vi "Run Time Register Data to Value Unit.vi"(0 "Value Reg Data":u16=1 caption="数值寄存器", 3 "Unit Reg Data":u16=100 caption="单位寄存器") -> (7 "Run Time Value":dbl=100.0 caption="运行时间值", 10 "Run Time Unit":string caption="运行时间单位")   [LabVIEW 2023, in "Longer Pump dLSP501 Series.lvlib"]
uses:
  <instrlib>/Longer Pump dLSP501 Modbus RTU Series/Longer Pump dLSP501 Series.lvlib
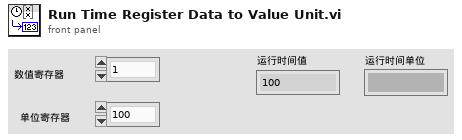
[diagram p1: front panel]
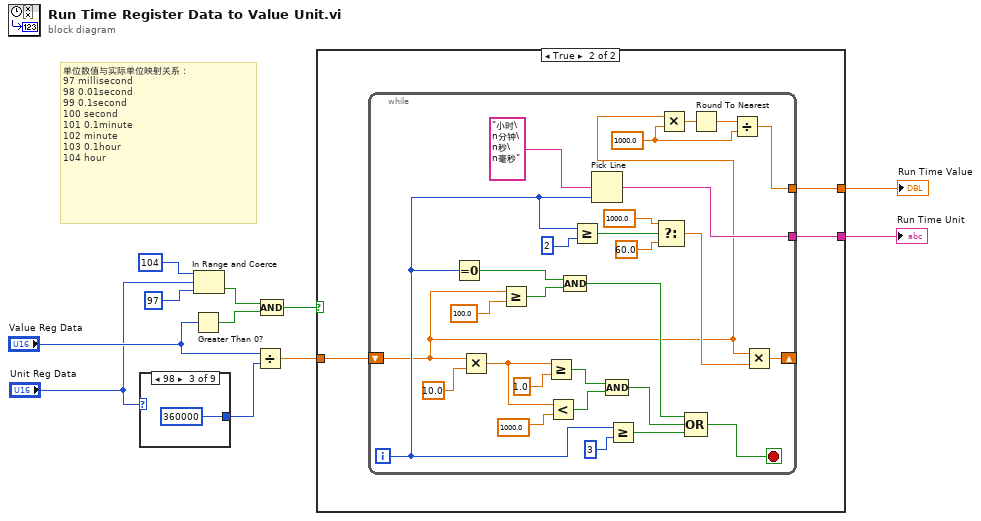
[diagram p0: block diagram]
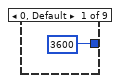
[diagram p2: hidden frame]
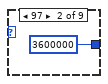
[diagram p3: hidden frame]
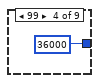
[diagram p4: hidden frame]
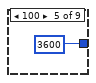
[diagram p5: hidden frame]
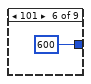
[diagram p6: hidden frame]
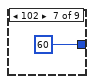
[diagram p7: hidden frame]
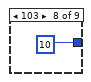
[diagram p8: hidden frame]
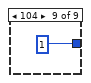
[diagram p9: hidden frame]
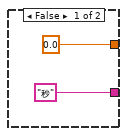
[diagram p10: hidden frame]
diagram:
  # "单位数值与实际单位映射关系：\n97\tmillisecond\n98\t0.01second\n99\t0.1second\n100\tsecond\n101\t0.1minute\n102\tminute\n103\t0.1hour\n104\thour"
  n1 = case shown="98" "Unit Reg Data" {
    tunnel: [3600 3600000 360000 36000 3600 600 60 10 1] -> w1
    frame 0, Default {
    }
    frame 97 {
    }
    frame 98 {
    }
    frame 99 {
    }
    frame 100 {
    }
    frame 101 {
    }
    frame 102 {
    }
    frame 103 {
    }
    frame 104 {
    }
  }
  n2 = Greater Than 0?(x="Value Reg Data") -> (x > 0?=w7:bool)
  n3 = In Range and Coerce(upper limit=u16 104 ("上限"), x="Unit Reg Data", lower limit=u16 97 ("下限")) -> (In Range?=w6:bool)  [unwired: 1 out]
  n4 = Divide(x="Value Reg Data", y=w1) -> (x/y=w10:dbl)
  n5 = Compound Arithmetic op=AND ("复合运算")(w6, w7) -> (w5:bool)
  n6 = case shown="True" w5 {
    tunnel: w10 -> [_ w25]
    tunnel: ["秒" w24] -> w9
    tunnel: [0.0 ("x") w23] -> w8
    frame False {
    }
    frame True {
      n7 = while {
        tunnel: [w42] -> w24
        tunnel: [w28] -> w23
        shift-right: [w41] -> _
        shift-left: w25 -> [w26]
        i -> [w36]
        stop <- w44 stop-if-true
        w27 = 1000.0 ("y")
        n8 = Equal To 0?(x=w36) -> (x = 0?=w39:bool)
        n9 = Multiply(x=w26, y=10.0 ("y 2")) -> (x*y=w51:dbl)
        n10 = Greater Or Equal?(x=w26, y=100.0 ("y 2")) -> (x >= y?=w38:bool)
        n11 = Greater Or Equal?(x=w51, y=1.0) -> (x >= y?=w49:bool)
        n12 = Less?(x=w51, y=1000.0) -> (x < y?=w48:bool)
        n13 = Compound Arithmetic op=AND ("复合运算")(w39, w38) -> (w37:bool)
        n14 = Greater Or Equal?(x=w36, y=2) -> (x >= y?=w34:bool)
        n15 = Pick Line(multi-line string="小时\n分钟\n秒\n毫秒", line index=w36) -> (output string=w42:string)  [unwired: 1 in]
        n16 = Compound Arithmetic op=AND ("复合运算")(w49, w48) -> (w45:bool)
        n17 = Greater Or Equal?(x=w36, y=3) -> (x >= y?=w46:bool)
        n18 = Select(t=1000.0 ("f"), s=w34, f=60.0) -> (s? t:f=w31:dbl)
        n19 = Multiply(x=w26, y=w27) -> (x*y=w30:dbl)
        n20 = Compound Arithmetic op=OR ("复合运算")(w37, w45, w46) -> (w44:bool)
        n21 = Round To Nearest(number=w30) -> (nearest integer value=w29:dbl)
        n22 = Divide(x=w29, y=w27) -> (x/y=w28:dbl)
        n23 = Multiply(x=w26, y=w31) -> (x*y=w41:dbl)
      }
    }
  }
  "Run Time Value" <- w8
  "Run Time Unit" <- w9
